vi "Warmup Unit of Work.vi"() -> (0 "error out":errorcluster)   [LabVIEW 2020, in "Conditu2.lvlib" / "Entity Manager.lvclass"]
uses:
  Entity Manager.lvclass
  Unit Of Work Session/Unit Of Work Session.lvclass
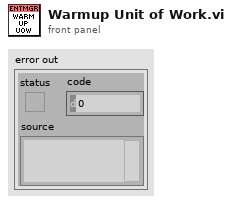
[diagram p1: front panel]
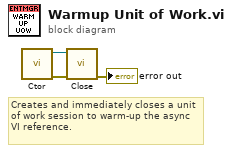
[diagram p0: block diagram]
diagram:
  # "Creates and immediately closes a unit of work session to warm-up the async VI reference."
  n1 = call "Ctor.vi"() -> ("error out"=w3:errorcluster, "Unit Of Work out"=w2:refnum<class "Unit Of Work Session.lvclass">)  [unwired: 10 in]
  n2 = call "Close.vi"("error in (no error)"=w3, "Unit Of Work in"=w2) -> ("error out"=→"error out":errorcluster)  [unwired: 9 in]
